vi "Solve2.vi"(8 "Error In":errorcluster, 11 "object in":refnum<class "2022_2.lvclass">) -> (0 "Error Out":errorcluster, 2 "Result":u64, 3 "object out":refnum<class "2022_2.lvclass">)   [LabVIEW 2020, in "2022_2.lvclass"]
uses:
  2022_2.lvclass
  2022_2.lvclass/2022_2.ctl
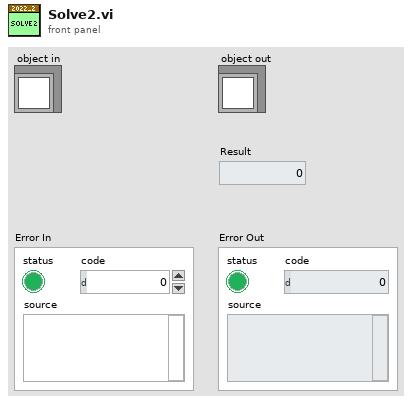
[diagram p1: front panel]
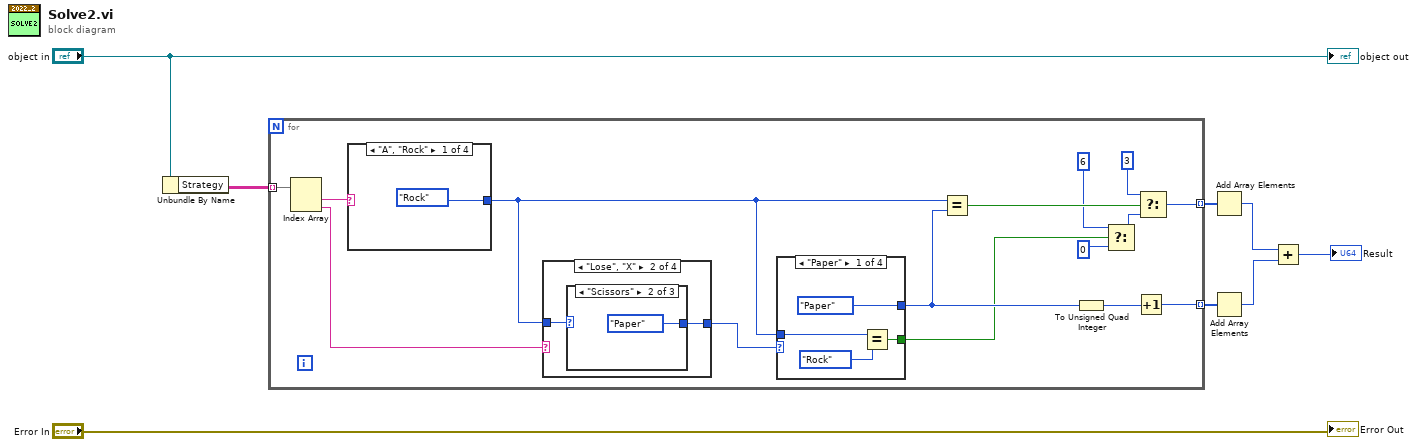
[diagram p0: block diagram]
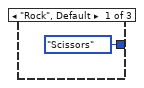
[diagram p3: hidden frame]
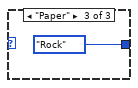
[diagram p4: hidden frame]
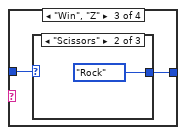
[diagram p5: hidden frame]
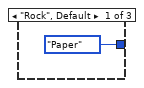
[diagram p6: hidden frame]
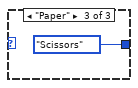
[diagram p7: hidden frame]
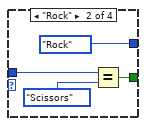
[diagram p9: hidden frame]
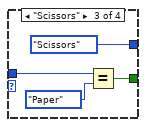
[diagram p10: hidden frame]
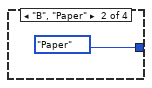
[diagram p12: hidden frame]
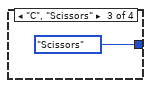
[diagram p13: hidden frame]
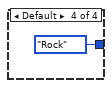
[diagram p14: hidden frame]
diagram:
  n1 = Unbundle By Name("object in") -> ("Strategy"=w2:string[][])
  n2 = for {
    tunnel: w2 -> [w23] mode=indexing
    tunnel: [w17] -> w6 mode=indexing
    tunnel: [w14] -> w4 mode=indexing
    n3 = Index Array(array=w23) -> (element #1=w22:string, element #2=w10:string)  [unwired: 2 in]
    n4 = case shown="\"A\", \"Rock\"" w22 {
      tunnel: [enum16{"Rock", "Paper", "Scissors"}."Rock" enum16{"Rock", "Paper", "Scissors"}."Paper" enum16{"Rock", "Paper", "Scissors"}."Scissors" enum16{"Rock", "Paper", "Scissors"}."Rock"] -> w11
      frame "A", "Rock" {
      }
      frame "B", "Paper" {
      }
      frame "C", "Scissors" {
      }
      frame Default {
      }
    }
    n5 = case shown="\"Lose\", \"X\"" w10 {
      tunnel: w11 -> [_ w25 w30 w34]
      tunnel: [_ w24 w29 w34] -> w9
      frame Default {
      }
      frame "Lose", "X" {
        n6 = case shown="\"Scissors\"" w25 {
          tunnel: [enum16{"Rock", "Paper", "Scissors"}."Scissors" enum16{"Rock", "Paper", "Scissors"}."Paper" enum16{"Rock", "Paper", "Scissors"}."Rock"] -> w24
          frame "Rock", Default {
          }
          frame "Scissors" {
          }
          frame "Paper" {
          }
        }
      }
      frame "Win", "Z" {
        n7 = case shown="\"Scissors\"" w30 {
          tunnel: [enum16{"Rock", "Paper", "Scissors"}."Paper" enum16{"Rock", "Paper", "Scissors"}."Rock" enum16{"Rock", "Paper", "Scissors"}."Scissors"] -> w29
          frame "Rock", Default {
          }
          frame "Scissors" {
          }
          frame "Paper" {
          }
        }
      }
      frame "Draw", "Y" {
      }
    }
    n8 = case shown="\"Paper\"" w9 {
      tunnel: [enum16{"Rock", "Paper", "Scissors"}."Paper" enum16{"Rock", "Paper", "Scissors"}."Rock" enum16{"Rock", "Paper", "Scissors"}."Scissors" _] -> w16
      tunnel: [w35 w39 w43 _] -> w13
      tunnel: w11 -> [w36 w41 w44 _]
      frame "Paper" {
        n9 = Equal?(x=w36, y=enum16{"Rock", "Paper", "Scissors"}."Rock") -> (x = y?=w35:bool)
      }
      frame "Rock" {
        n10 = Equal?(x=w41, y=enum16{"Rock", "Paper", "Scissors"}."Scissors") -> (x = y?=w39:bool)
      }
      frame "Scissors" {
        n11 = Equal?(x=w44, y=enum16{"Rock", "Paper", "Scissors"}."Paper") -> (x = y?=w43:bool)
      }
      frame Default {
      }
    }
    n12 = Equal?(x=w11, y=w16) -> (x = y?=w21:bool)
    n13 = To Unsigned Quad Integer(1:w16) -> (0:w15:u64)
    n14 = Select(t=u64 6, s=w13, f=u64 0) -> (s? t:f=w18:u64)
    n15 = Increment(x=w15) -> (x+1=w14:u64)
    n16 = Select(t=u64 3, s=w21, f=w18) -> (s? t:f=w17:u64)
  }
  n17 = Add Array Elements(numeric array=w6) -> (sum=w5:u64)
  n18 = Add Array Elements(numeric array=w4) -> (sum=w3:u64)
  n19 = Add(x=w5, y=w3) -> (x+y=→"Result":u64)
  "Error Out" <- "Error In"
  "object out" <- "object in"
